vi "Acquire Status.vi"(8 "error in (no error)":errorcluster, 11 "DAQ DI in":refnum<class "DAQ DI.lvclass">) -> (0 "error out":errorcluster, 3 "DAQ DI out":refnum<class "DAQ DI.lvclass">)   [LabVIEW 2020, in "DAQ DI.lvlib" / "DAQ DI.lvclass"]
uses:
  DAQ DI.lvclass
  DAQ DI.lvclass/DAQ DI.ctl
  <vilib>/DAQmx/read.llb/DAQmx Read (Digital U8 1Chan 1Samp).vi
  <vilib>/numeric/Random Number (Range) U64.vi
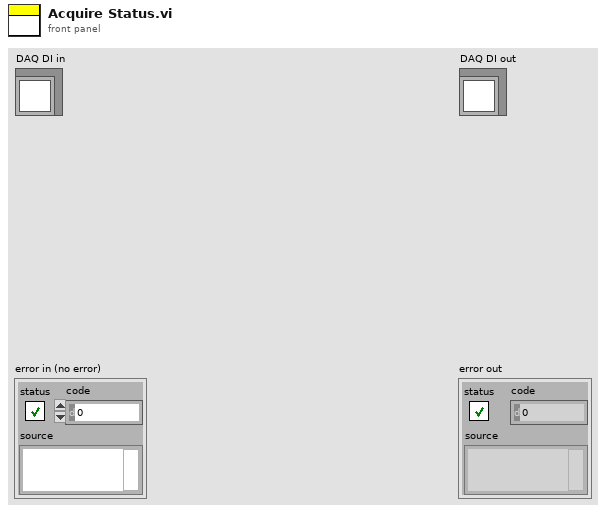
[diagram p1: front panel]
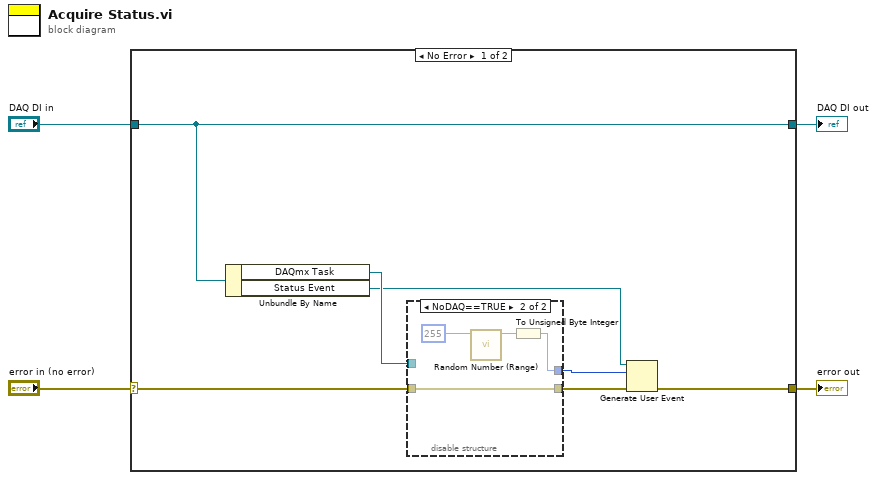
[diagram p0: block diagram]
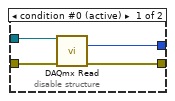
[diagram p2: hidden frame]
diagram:
  n1 = case shown="No Error" "error in (no error)" {
    selector: "error in (no error)" -> [w9 w21]
    tunnel: [w5 w21] -> w3
    tunnel: [w11 w20] -> w1
    tunnel: "DAQ DI in" -> [w11 w20]
    frame No Error {
      n2 = Unbundle By Name(w11) -> ("DAQmx Task"=w10:refnum<k21>, "Status Event"=w8:refnum<user-event>)
      n3 = disable-structure shown="NoDAQ==TRUE" {
        disable-tunnel: w10 -> [w15 _]
        disable-tunnel: w9 -> [w14 w19]
        disable-tunnel: [w13 w16] -> w7
        disable-tunnel: [w12 w19] -> w6
        frame condition #0 (active) {
          n4 = call-poly <vilib>:"DAQmx Read.vi"("task/channels in"=w15, "error in"=w14) -> ("data"=w13:u8, "error out"=w12:errorcluster)  [unwired: 11 in, 1 out]
        }
        frame condition #1 {
          n5 = call-poly <vilib>:"Random Number (Range).vi"("upper bound (100)"=u64 255) -> ("number"=w17:u64)  [unwired: 10 in]
          n6 = To Unsigned Byte Integer(number=w17) -> (unsigned 8bit integer=w16:u8)
        }
      }
      n7 = Generate User Event(user event=w8, event data cluster=w7, error in=w6) -> (error out=w5:errorcluster)  [unwired: 1 in, 1 out]
    }
    frame Error {
    }
  }
  "error out" <- w3
  "DAQ DI out" <- w1
